vi "Actor Core.vi"(8 "error in":errorcluster, 11 "Network Stream Reader in":refnum<class "Network Stream Reader.lvclass">) -> (0 "error out":errorcluster, 3 "Actor out":refnum<class "Actor.lvclass">)   [LabVIEW 2014, in "Network Stream Reader.lvlib" / "Network Stream Reader.lvclass"]
doc: "(<B>Filename</B>: Actor Framework.lvlib:Actor.lvclass:Actor Core.vi)\n\nReceives messages to the actor, reacts to them, and initiates any error handling that may shut the actor down.\n\nDescendant classes may override this VI to append parallel tasks for the actor to complete while it handles messages. Overrides use the Call Parent Method node."
uses:
  Network Stream Reader.lvclass
  <vilib>/ActorFramework/Actor/Actor.lvclass
  Network Stream Reader.lvclass/Network Stream Reader.ctl
  Proxy/Proxy/Proxy.lvclass/Proxy.ctl
  <vilib>/ActorFramework/Actor/Actor.lvclass/Actor.ctl
  Network Stream/Network Stream/Network Stream.lvclass/Network Stream.ctl
  <vilib>/ActorFramework/Message Enqueuer/Message Enqueuer.lvclass/Message Enqueuer.ctl
  Network Stream/Network Stream/MessageString.ctl
  <vilib>/ActorFramework/Message Enqueuer/Message Priority.ctl
  <vilib>/ActorFramework/Stop Msg/Stop Msg.lvclass/Stop Msg.ctl
  Proxy/Proxy/Read Target Enq.vi
  Network Stream/Network Stream/Read timeout.vi
  Network Stream/Network Stream/Read Buffer Size.vi
  Network Stream/Network Stream/Read Context.vi
  Network Stream/Network Stream/Read Name.vi
  <vilib>/ActorFramework/Message Enqueuer/Init from Existing Queue.vi
  <vilib>/ActorFramework/Stop Msg/Send Emergency Stop.vi
  <vilib>/ActorFramework/Stop Msg/Send Normal Stop.vi
  <vilib>/ActorFramework/Message Enqueuer/Equals Not A Refnum.vi
  <vilib>/ActorFramework/Actor/Read Caller Enqueuer.vi
  <vilib>/ActorFramework/Message Enqueuer/Enqueue Critical.vi
  <vilib>/ActorFramework/Message Priority Queue/Priority Enqueue.vi
  Network Stream/Network Stream/Network Stream.lvclass
  <vilib>/ActorFramework/Message Enqueuer/Message Enqueuer.lvclass
  <vilib>/ActorFramework/Stop Msg/Stop Msg.lvclass
  <resource>/objmgr/ni.dex.rc
panel:
  out "Is Connected":bool
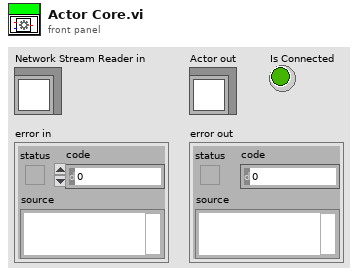
[diagram p1: front panel]
types:
  T1 = typedef "Network Stream.lvlib/Network Stream.lvclass/MessageString.ctl" = cluster{"Flatten Msg":string, "Message Priority":T2}
  T2 = typedef "Actor Framework.lvlib/Message Enqueuer.lvclass/Message Priority.ctl" = enum16{"Low", "Normal", "High"}
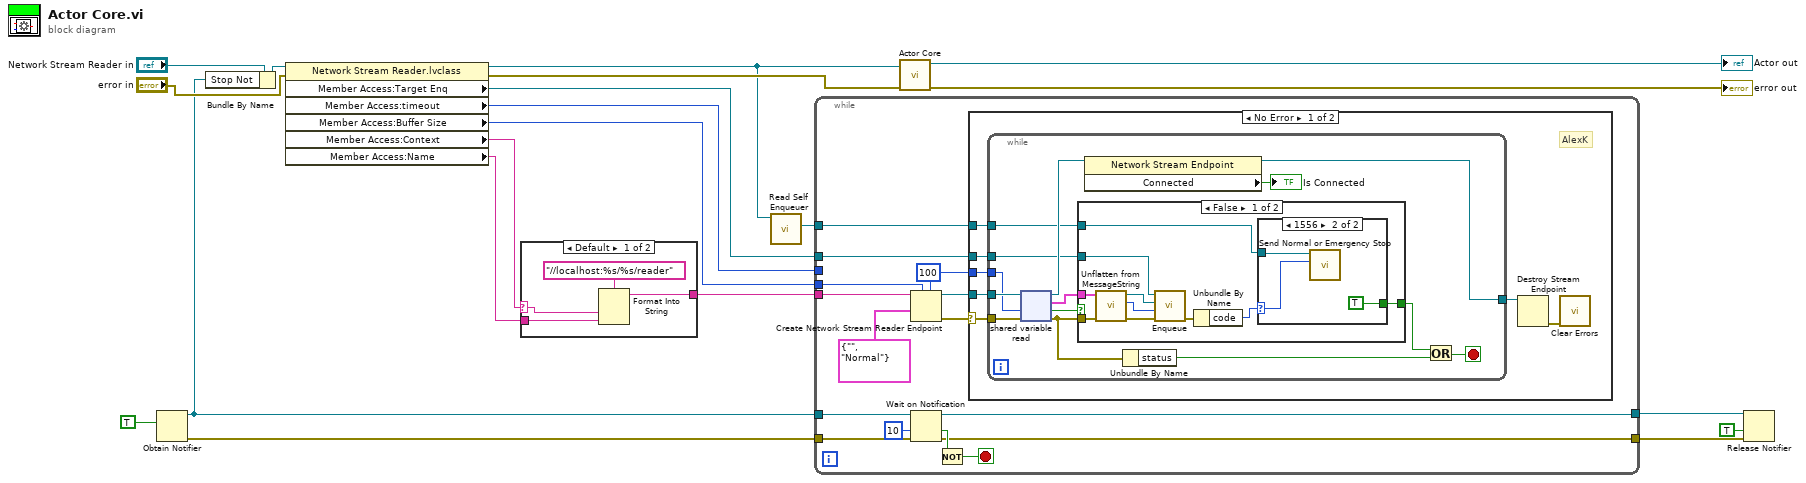
[diagram p0: block diagram]
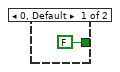
[diagram p2: hidden frame]
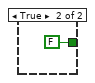
[diagram p3: hidden frame]
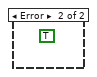
[diagram p4: hidden frame]
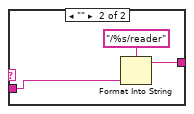
[diagram p5: hidden frame]
diagram:
  n1 = Obtain Notifier(notification data type=TRUE) -> (notifier out=w5:refnum<notifier>, error out=w4:errorcluster)  [unwired: 3 in, 1 out]
  n2 = Bundle By Name(cluster="Network Stream Reader in", "Stop Not"=w5) -> (w6:refnum<class "Network Stream Reader.lvclass">)
  n3 = property on="Property Node" class="Network Stream Reader.lvclass"(reference=w6, error in="error in") -> (reference out=w2:refnum<class "Network Stream Reader.lvclass">, error out=w12:errorcluster, "Member Access:Target Enq"=w18:refnum<class "Message Enqueuer.lvclass">, "Member Access:timeout"=w17:i32, "Member Access:Buffer Size"=w16:i32, "Member Access:Context"=w14:string, "Member Access:Name"=w13:string)
  n4 = case shown="Default" w14 {
    selector: w14 -> [w21 _]
    tunnel: [w23 w26] -> w11
    tunnel: w13 -> [w22 w25]
    frame Default {
      n5 = Format Into String(format string="//localhost:%s/%s/reader", w21, w22) -> (resulting string=w23:string)  [unwired: 2 in, 1 out]
    }
    frame "" {
      n6 = Format Into String(format string="/%s/reader", w25) -> (resulting string=w26:string)  [unwired: 2 in, 1 out]
    }
  }
  n7 = call <vilib>:"Read Self Enqueuer.vi"("Actor"=w2) -> ("Self Enqueuer"=w1:refnum<class "Message Enqueuer.lvclass">)  [unwired: 10 in]
  n8 = while {
    tunnel: w18 -> [w42]
    tunnel: w17 -> [_]
    tunnel: w16 -> [w41]
    tunnel: w11 -> [w38]
    tunnel: w5 -> [w36]
    tunnel: [w35] -> w8
    tunnel: w4 -> [w32]
    tunnel: [w31] -> w3
    tunnel: w1 -> [w28]
    stop <- w33 stop-if-true
    w37 = 100 ("timeout in ms (-1)")
    n9 = Create Network Stream Reader Endpoint(5:w37, 7:w41, 9:T1 {"Flatten Msg"="", "Message Priority"=enum."Normal"} ("Msg String"), 11:w38) -> (0:w39:errorcluster, 3:w40:refnum<k21>)  [unwired: 3 in]
    n10 = Wait on Notification(notifier=w36, timeout in ms (-1)=10, error in (no error)=w32) -> (notifier out=w35:refnum<notifier>, timed out?=w34:bool, error out=w31:errorcluster)  [unwired: 1 in, 1 out]
    n11 = Not(x=w34) -> (.not. x?=w33:bool)
    n12 = case shown="No Error" w39 {
      selector: w39 -> [w48 _]
      tunnel: w42 -> [w45 _]
      tunnel: w40 -> [w47 _]
      tunnel: w37 -> [w44 _]
      tunnel: w28 -> [w43 _]
      frame No Error {
        # "AlexK"
        n13 = while {
          tunnel: w48 -> [w63]
          tunnel: w47 -> [w61]
          tunnel: [w56] -> w49
          tunnel: w45 -> [w59]
          tunnel: w44 -> [w57]
          tunnel: w43 -> [w50]
          stop <- w52 stop-if-true
          n14 = shared-variable-read(w61, w63, w57) -> (w60:refnum<k21>, w54:errorcluster, w58:bool, w62:T1)
          n15 = case shown="False" w58 {
            tunnel: w62 -> [w72 _]
            tunnel: w59 -> [w73 _]
            tunnel: w54 -> [w68 _]
            tunnel: [w65 FALSE] -> w51
            tunnel: w50 -> [w64 _]
            frame False {
              n16 = call "Unflatten from MessageString.vi"("error in (no error)"=w68, "Msg String"=w72) -> ("error out"=w69:errorcluster, "Message Priority"=w70:T2, "Actor Framework:Message"=w71:refnum<class "Message.lvclass">)  [unwired: 7 in]
              n17 = call <vilib>:"Enqueue.vi"("error in (no error)"=w69, "Message Priority (Normal)"=w70, "Message"=w71, "Message Enqueuer in"=w73) -> ("error out"=w67:errorcluster)  [unwired: 6 in, 1 out]
              n18 = Unbundle By Name(w67) -> ("code"=w66:i32)
              n19 = case shown="1556" w66 {
                selector: w66 -> [_ w75]
                tunnel: [FALSE TRUE] -> w65
                tunnel: w64 -> [_ w76]
                frame 0, Default {
                }
                frame 1556 {
                  n20 = call <vilib>:"Send Normal or Emergency Stop.vi"("final error code"=w75, "Message Enqueuer"=w76) -> ()  [unwired: 9 in, 1 out]
                }
              }
            }
            frame True {
            }
          }
          n21 = property class="Network Stream Endpoint"(reference=w60) -> (reference out=w56:refnum<k21>, "Connected"=→"Is Connected":bool)  [unwired: 1 in, 1 out]
          n22 = Unbundle By Name(w54) -> ("status"=w53:bool)
          n23 = Or(x=w51, y=w53) -> (x .or. y?=w52:bool)
        }
        n24 = Destroy Stream Endpoint(11:w49) -> (0:w46:errorcluster)  [unwired: 1 in]
        n25 = call <vilib>:"Clear Errors.vi"("error in (no error)"=w46) -> ()  [unwired: 5 in, 2 out]
      }
      frame Error {
        (unwired) TRUE
      }
    }
  }
  n26 = call-parent "Actor Core.vi"("error in"=w12, "Actor in"=w2) -> ("error out"=→"error out":errorcluster, "Actor out"=→"Actor out":refnum<class "Actor.lvclass">)  [unwired: 8 in]
  n27 = Release Notifier(notifier=w8, force destroy? (F)=TRUE, error in (no error)=w3) -> ()  [unwired: 3 out]
